vi "Create.vi"(8 "error in (no error)":errorcluster, 10 "Input":string) -> (0 "error out":errorcluster, 3 "Proto":refnum<class "Maze.lvclass">)   [LabVIEW 2021, in "Maze.lvclass"]
uses:
  Maze.lvclass
  Maze.lvclass/Maze.ctl
  Helpers/Helpers.lvlib
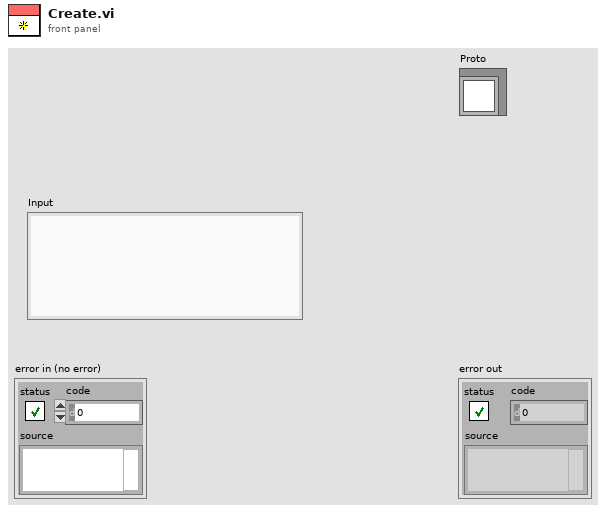
[diagram p1: front panel]
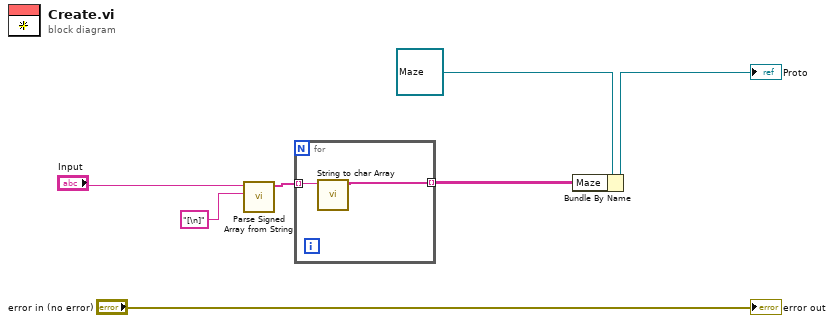
[diagram p0: block diagram]
diagram:
  n1 = call "Parse Signed Array from String.vi"("Delimiter regex"="[\n]", "Input"="Input") -> ("Parsed Array"=w3:string[])  [unwired: 8 in, 1 out]
  n2 = for {
    tunnel: w3 -> [w9] mode=indexing
    tunnel: [w8] -> w1 mode=indexing
    n3 = call "String to char Array.vi"("Row"=w9) -> ("Array"=w8:string[])  [unwired: 10 in]
  }
  n4 = Bundle By Name(cluster=refnum<class "Maze.lvclass"> refnum ("Proto"), "Maze"=w1) -> (→"Proto":refnum<class "Maze.lvclass">)
  "error out" <- "error in (no error)"
